vi "ArrayToXYGraph.vi"(0 "input array":dbl[][](array[numeric]), 1 "\"row\" or \"col\"":string, 2 "row or col index for X data":i32, 3 "row or col index for Y data":i32) -> (6 "cluster for XY graph":cluster{"array":dbl[], "array":dbl[]})   [LabVIEW 2015]
doc: "Takes a 2d array and prepares it to use as input for an XY graph. Specifically, takes either 2 rows or 2 columns of the array (depending whether \"row\" or \"col\" is indicated) and bundles them together into a cluster."
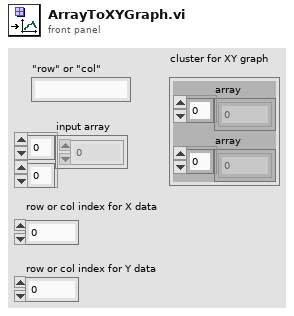
[diagram p1: front panel]
types:
  T1 = cluster{"input array":dbl[], "input array":dbl[]}
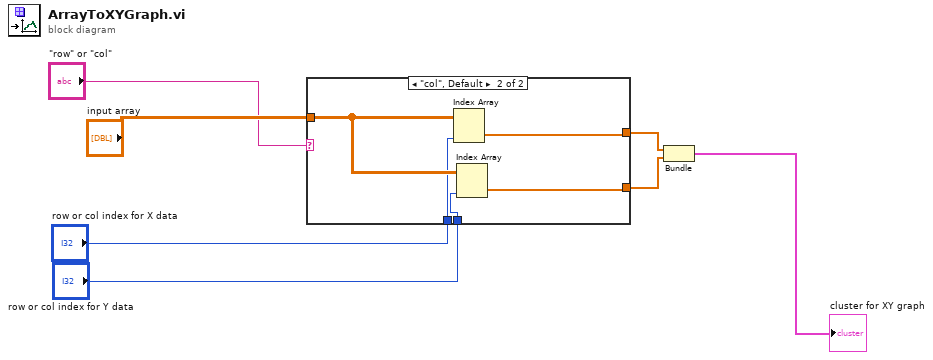
[diagram p0: block diagram]
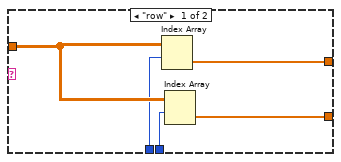
[diagram p2: hidden frame]
diagram:
  n1 = case shown="\"col\", Default" "\"row\" or \"col\"" {
    tunnel: "input array" -> [w12 w17]
    tunnel: "row or col index for X data" -> [w11 w16]
    tunnel: "row or col index for Y data" -> [w10 w15]
    tunnel: [w9 w14] -> w6
    tunnel: [w8 w13] -> w7
    frame "row" {
      n2 = Index Array(array=w12, index (row)=w11) -> (element=w9:dbl[])  [unwired: 1 in]
      n3 = Index Array(array=w12, index (row)=w10) -> (element=w8:dbl[])  [unwired: 1 in]
    }
    frame "col", Default {
      n4 = Index Array(array=w17, index (col)=w16) -> (element=w14:dbl[])  [unwired: 1 in]
      n5 = Index Array(array=w17, index (col)=w15) -> (element=w13:dbl[])  [unwired: 1 in]
    }
  }
  n6 = Bundle("input array"=w6, "input array"=w7) -> (→"cluster for XY graph":T1)  [unwired: 1 in]
